vi "time_frame.vi"() -> ()   [LabVIEW 2017]
panel:
  in  "felharmonikus N":i32=2
  in  "SNR window width [Hz]":dbl=0.4 format="%#_13g"
  in  "Case select":string(combo)
  out "mean":cluster{"X":dbl, "Y":dbl}[](graph)
  out "szum":cluster{"X":dbl, "Y":dbl}[](graph)
  out "sd":cluster{"X":dbl, "Y":dbl}[](graph)
  out "szum/time":cluster{"X":dbl, "Y":dbl}[](graph)
  out "X SNR 3 (bigger better)":cluster{"X":dbl, "Y":dbl}[](graph)
  out "X SNR 4":cluster{"X":dbl, "Y":dbl}[](graph)
  out "X SNR":cluster{"X":dbl, "Y":dbl}[](graph)
  in  "Path":path=path "C:/Users/Lenovo/Desktop/szakdoga/data/time"
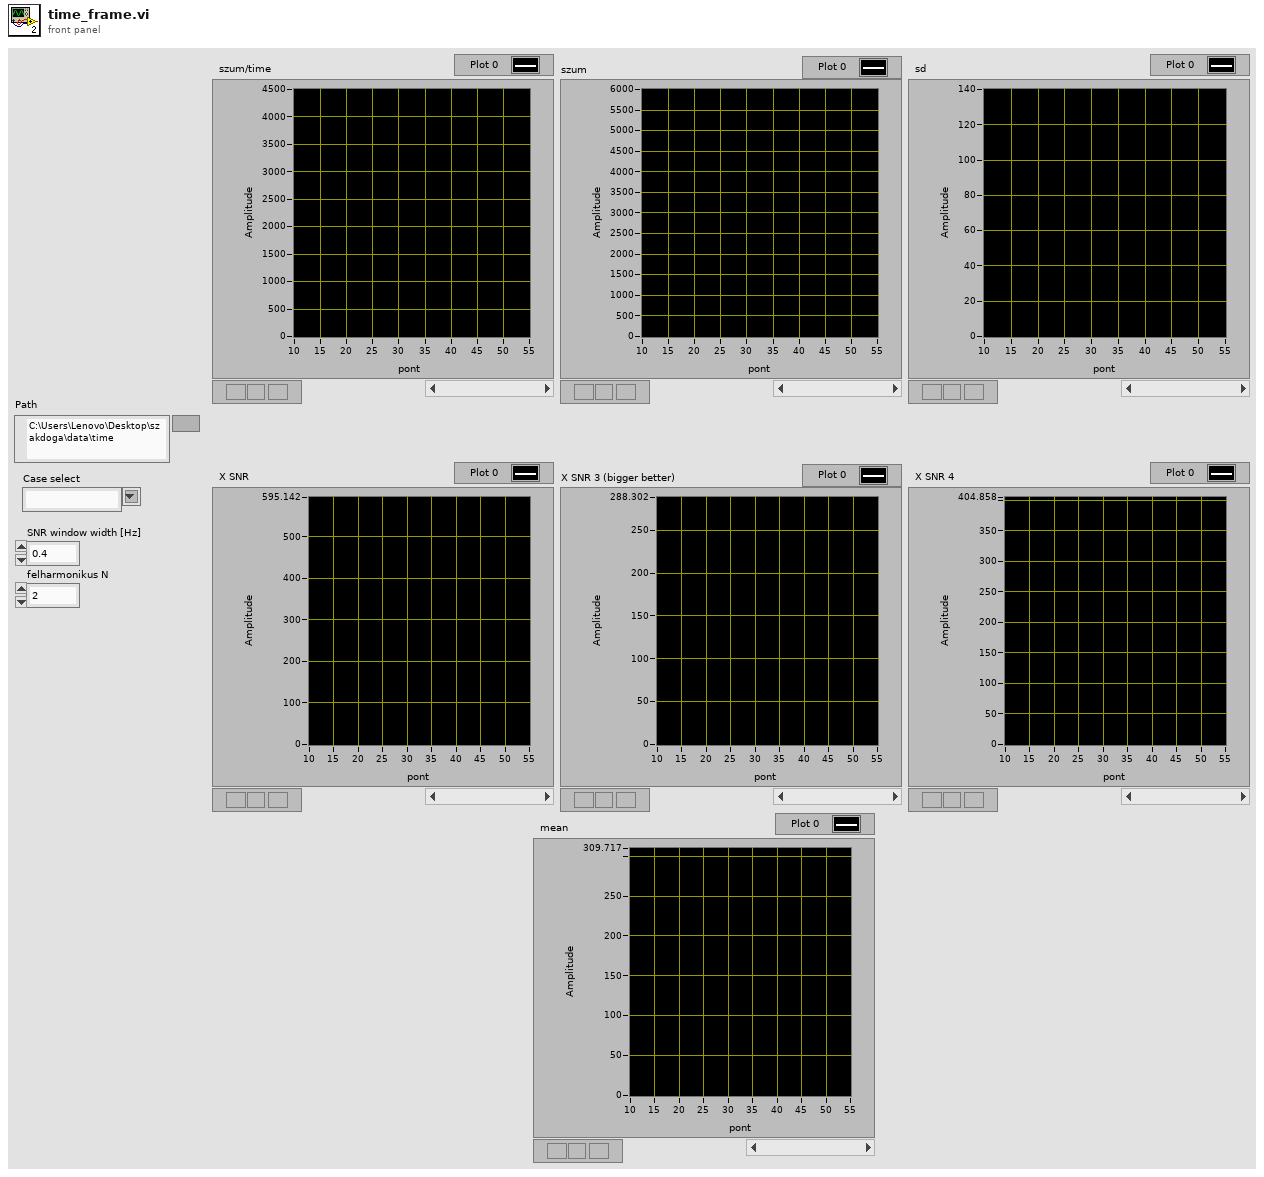
[diagram p1: front panel]
types:
  T1 = cluster{cluster{dbl, "impulse szum/time":dbl}[], cluster{dbl, "impulse  szum":dbl}[], cluster{dbl, "impulse standard deviation":dbl}[], cluster{dbl, "impulse mean":dbl}[], cluster{dbl, "X SNR 1":dbl}[], cluster{dbl, "X SNR 2":dbl}[], cluster{dbl, "X SNR 3":dbl}[]}
  T2 = cluster{cluster{dbl, "impulse szum/time":dbl}[], cluster{dbl, "impulse  szum":dbl}[], cluster{dbl, "impulse standard deviation":dbl}[], cluster{dbl, "impulse mean":dbl}[], cluster{dbl, "X SNR 1":dbl}[], cluster{dbl, "X SNR 2":dbl}[], cluster{dbl, "X SNR 3":dbl}[], cluster{dbl, "impulse szum/avg":dbl}[]}
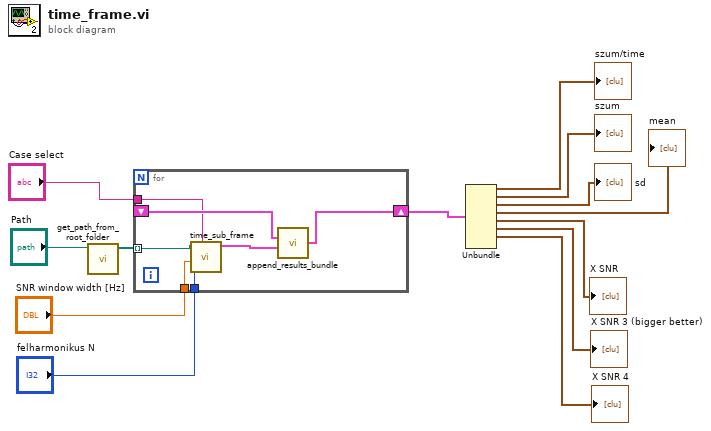
[diagram p0: block diagram]
diagram:
  n1 = call "get_path_from_root_folder.vi"("Path"="Path") -> ("Array"=w12:path[])  [unwired: 9 in, 1 out]
  n2 = for {
    shift-right: [w19] -> w13
    shift-left: _ -> [w20]
    tunnel: w12 -> [w18] mode=indexing
    tunnel: "Case select" -> [w16]
    tunnel: "SNR window width [Hz]" -> [w15]
    tunnel: "felharmonikus N" -> [w14]
    n3 = call "time_sub_frame.vi"("Case select"=w16, "felharmonikus N"=w14, "SNR window width [Hz]"=w15, "path to binary file"=w18) -> ("output cluster"=w17:T1)  [unwired: 7 in]
    n4 = call "append_results_bundle.vi"("Y"=w17, "X"=w20) -> ("concat(X,Y)"=w19:T2)  [unwired: 8 in]
  }
  n5 = Unbundle(w13) -> (→"szum/time":cluster{dbl, "impulse szum/time":dbl}[], →"szum":cluster{dbl, "impulse  szum":dbl}[], →"sd":cluster{dbl, "impulse standard deviation":dbl}[], →"mean":cluster{dbl, "impulse mean":dbl}[], →"X SNR":cluster{dbl, "X SNR 1":dbl}[], →"X SNR 3 (bigger better)":cluster{dbl, "X SNR 2":dbl}[], →"X SNR 4":cluster{dbl, "X SNR 3":dbl}[])  [unwired: 1 out]
